vi "GT Get Capture Mode.vi"(7 "count":i16, 8 "error in (no error)":errorcluster caption="错误输入（无错误）", 9 "pMode":i16[](array[numeric]), 10 "encoder":i16, 11 "cardNum":i16) -> (0 "error out":errorcluster caption="错误输出", 1 "pMode out":i16[](array[numeric]), 3 "function return":i16)   [LabVIEW 2014, in "gts.lvlib"]
doc: "GT_API GT_GetCaptureMode(short cardNum,short encoder,short *pMode,short count=1);"
uses:
  gts.lvlib
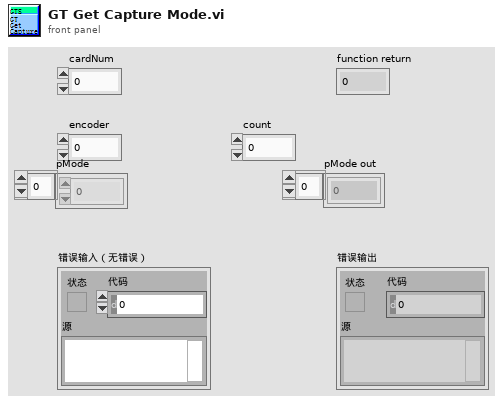
[diagram p1: front panel]
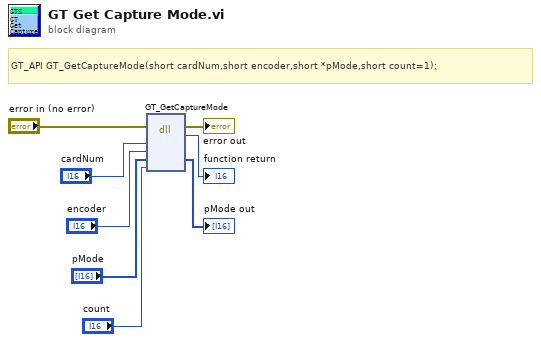
[diagram p0: block diagram]
diagram:
  # "GT_API GT_GetCaptureMode(short cardNum,short encoder,short *pMode,short count=1);"
  n1 = dll-call lib="PTH2habs D固高科技资料GTS控制卡GTS卡18年上半年资料dllVC32bit\nmulti_cardgts.*" fn="GT_GetCaptureMode"(error in="error in (no error)", "cardNum"="cardNum", "encoder"="encoder", "pMode"="pMode", "count"="count") -> (error out=→"error out":errorcluster, "返回类型"=→"function return":i16, "pMode"=→"pMode out":i16[])  [unwired: 5 in, 1 out]
